vi "Open LV-Proto Library.vi"(7 "App Refnum":refnum<vi>, 8 "error in (no error)":errorcluster) -> (0 "error out":errorcluster, 1 "VIs":refnum<vi>[](array[refnum]), 2 "Libraries":refnum<vi>[](array[refnum]), 3 "Library":refnum<vi>)   [LabVIEW 2020, in "LV-Protoc.lvlib"]
uses:
  LV-Protoc.lvlib
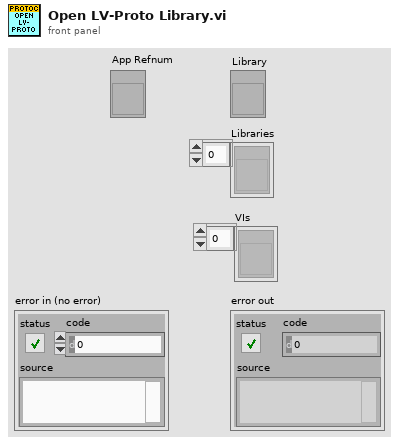
[diagram p1: front panel]
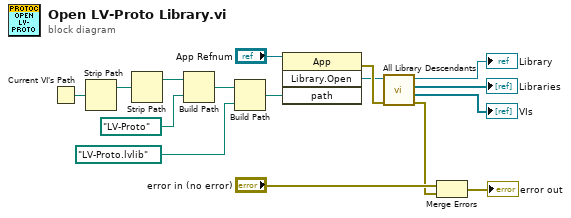
[diagram p0: block diagram]
diagram:
  n1 = Current VI's Path() -> (path=w15:path)
  n2 = Strip Path(path=w15) -> (stripped path=w14:path)  [unwired: 1 out]
  n3 = Strip Path(path=w14) -> (stripped path=w13:path)  [unwired: 1 out]
  n4 = Build Path(base path=w13, name or relative path=path "LV-Proto") -> (appended path=w11:path)
  n5 = Build Path(base path=w11, name or relative path=path "LV-Proto.lvlib") -> (appended path=w8:path)
  n6 = invoke class="App" method="Library.Open"(reference="App Refnum", "path"=w8) -> (error out=w16:errorcluster, "Open Library"=w7:refnum<vi>)  [unwired: 2 in, 2 out]
  n7 = call "All Library Descendants.vi"("error in (no error)"=w16, "Library in"=w7) -> ("error out"=w2:errorcluster, "VIs"=→"VIs":refnum<vi>[], "Libraries"=→"Libraries":refnum<vi>[], "Library"=→"Library":refnum<vi>)  [unwired: 6 in]
  n8 = Merge Errors("error in (no error)", w2) -> (→"error out":errorcluster)
